vi "current monitor.vi"() -> ()   [LabVIEW 2010]
uses:
  <vilib>/Utility/file.llb/Write To Spreadsheet File (DBL).vi
  <userlib>/Nanonis Prog Interface V5/Nanonis Prog Interface.lvlib
panel:
  in  "Convert to nm/s?":bool caption="Spectrum Analyzer 2"
  out "Spectrum Analyzer 2":cluster{"f0":dbl, "df":dbl, "values":dbl[]}(graph)
  in  "Spectrum Analyzer2":bool caption="Spectrum Analyzer 2"
  out "error out":errorcluster
  in  "Path":path
  out "Spectrum Analyzer":cluster{"f0":dbl, "df":dbl, "values":dbl[]}(graph)
  out "Current (A)":sgl format="%#_6p"
  out "Current":cluster{"Current (A)":dbl, dbl}[](graph)
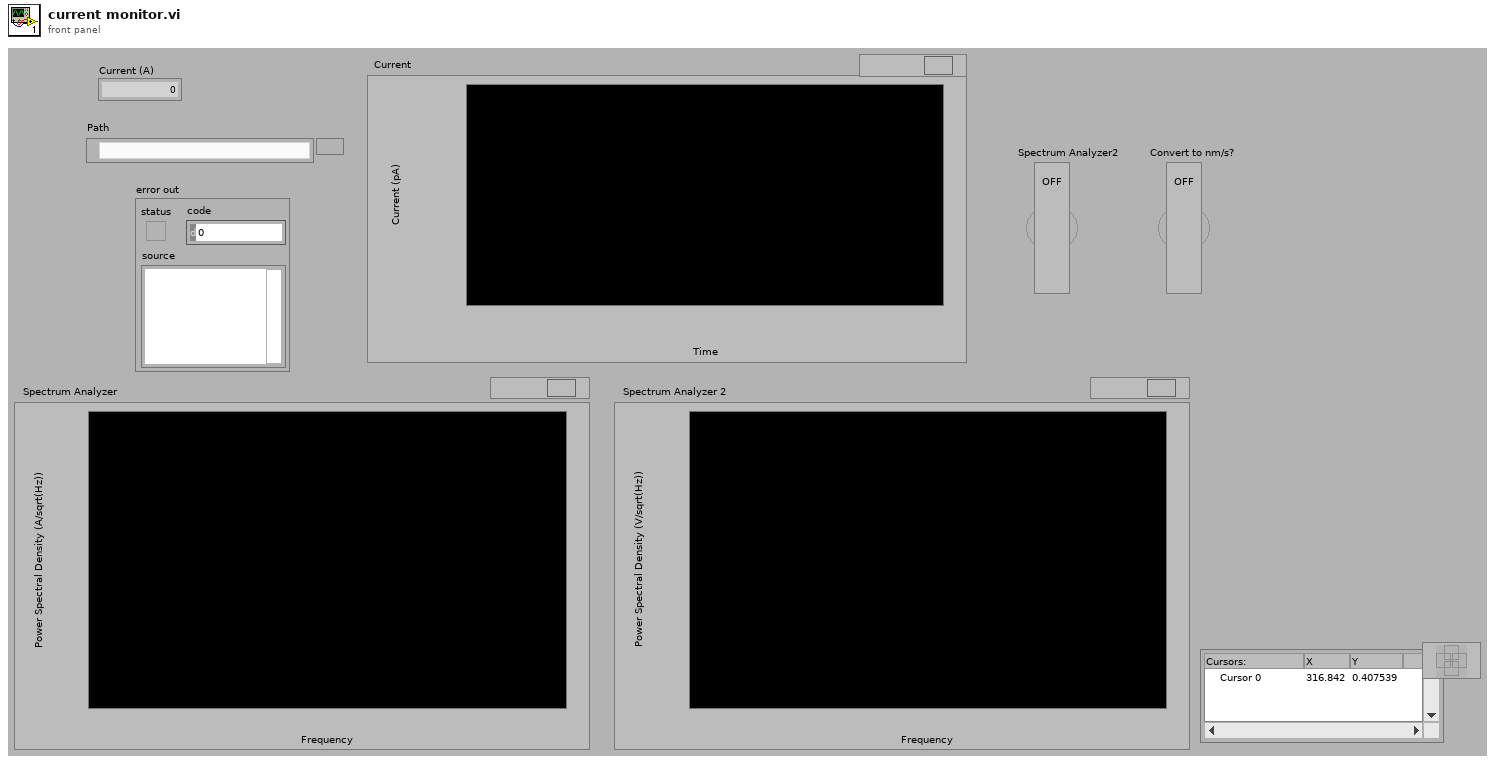
[diagram p1: front panel]
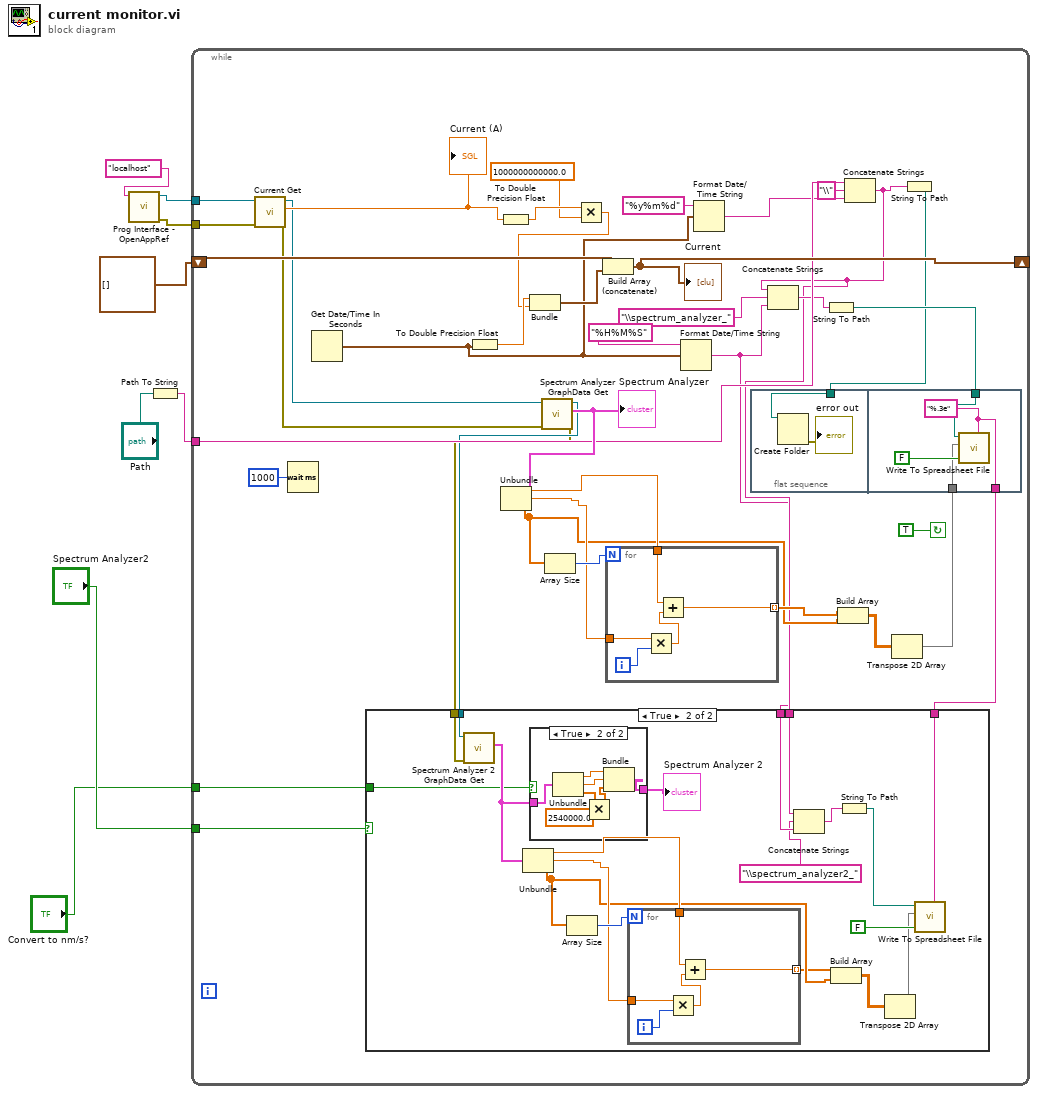
[diagram p0: block diagram]
diagram:
  n1 = call <userlib>:"Prog Interface - OpenAppRef.vi"("Machine name (local machine IP)"="localhost" ("machine name (localhost)")) -> ("Error out"=w7:errorcluster, "Application reference"=w8:refnum<vi>)  [unwired: 5 in]
  n2 = Path To String(path="Path") -> (string=w3:string)
  n3 = while {
    tunnel: w8 -> [w46]
    tunnel: w7 -> [w45]
    shift-right: [w42] -> _
    shift-left: cluster{dbl, dbl}[] [] -> [w43]
    tunnel: w3 -> [w28]
    tunnel: "Spectrum Analyzer2" -> [w13]
    tunnel: "Convert to nm/s?" -> [w9]
    stop <- TRUE continue-if-true
    n4 = call <userlib>:"Current Get.vi"("Error in (no error)"=w45, "Application ref in"=w46) -> ("Error out"=w35:errorcluster, "Current (A)"=w40:sgl, "Application ref out"=w36:refnum<vi>)  [unwired: 5 in]
    "Current (A)" <- w40
    n5 = Wait (ms)(milliseconds to wait=u32 1000) -> ()  [unwired: 1 out]
    n6 = Get Date/Time In Seconds() -> (seconds since 1Jan1904=w29:timestamp)
    n7 = To Double Precision Float(number=w29) -> (double precision float=w41:dbl)
    n8 = To Double Precision Float(number=w40) -> (double precision float=w39:dbl)
    n9 = call <userlib>:"Spectrum Analyzer GraphData Get.vi"("Error in (no error)"=w35, "Application ref in"=w36) -> ("Error out"=w14:errorcluster, "FFT data"=w33:cluster{"f0":dbl, "df":dbl, "values":dbl[]}, "Application ref out"=w15:refnum<vi>)  [unwired: 7 in]
    "Spectrum Analyzer" <- w33
    n10 = Unbundle(w33) -> ("f0"=w21:dbl, "df"=w20:dbl, "values"=w18:dbl[])
    n11 = Array Size(array=w18) -> (size(s)=w22:i32)
    n12 = Multiply(x=w39, y=1000000000000.0) -> (x*y=w38:dbl)
    n13 = Bundle(w41, w38) -> (w44:cluster{dbl, dbl})  [unwired: 1 in]
    n14 = Build Array (concatenate)(w43, w44) -> (w42:cluster{dbl, dbl}[])
    "Current" <- w42
    n15 = for {
      N: w22 -> [_]
      tunnel: w21 -> [w84]
      tunnel: w20 -> [w81]
      tunnel: [w80] -> w19 mode=indexing
      i -> [w82]
      n16 = Multiply(x=w81, y=w82) -> (x*y=w83:dbl)
      n17 = Add(x=w84, y=w83) -> (x+y=w80:dbl)
    }
    n18 = Format Date/Time String(time format string (%c)="%H%M%S", seconds (now)=w29) -> (date/time string=w11:string)  [unwired: 1 in]
    n19 = Format Date/Time String(time format string (%c)="%y%m%d", seconds (now)=w29) -> (date/time string=w26:string)  [unwired: 1 in]
    n20 = flat-sequence {
      tunnel: w27 -> [w86]
      tunnel: w31 -> [w88]
      tunnel: w16 -> [w89]
      tunnel: [w87] -> w10
      frame #0 {
        n21 = Create Folder(path (use dialog)=w86) -> (error out=→"error out":errorcluster)  [unwired: 2 in, 2 out]
      }
      frame #1 {
        w87 = "%.3e" ("format (%.3f)")
        n22 = call-poly <vilib>:"Write To Spreadsheet File.vi"("format (%.3f)"=w87, "append to file? (new file:F)"=FALSE, "2D data"=w89, "file path (dialog if empty)"=w88) -> ()  [unwired: 4 in, 1 out]
      }
    }
    n23 = Build Array(w19, w18) -> (w17:dbl[][])
    n24 = Concatenate Strings(w28, "\\" ("string"), w26) -> (w12:string)
    n25 = case shown="True" w13 {
      tunnel: w15 -> [_ w66]
      tunnel: w14 -> [_ w65]
      tunnel: w12 -> [_ w56]
      tunnel: w11 -> [_ w55]
      tunnel: w10 -> [_ w51]
      tunnel: w9 -> [_ w48]
      frame False {
      }
      frame True {
        n26 = call <userlib>:"Spectrum Analyzer 2 GraphData Get.vi"("Error in (no error)"=w65, "Application ref in"=w66) -> ("FFT data"=w50:cluster{"f0":dbl, "df":dbl, "values":dbl[]})  [unwired: 7 in, 2 out]
        n27 = Unbundle(w50) -> ("f0"=w63:dbl, "df"=w62:dbl, "values"=w60:dbl[])
        n28 = case shown="True" w48 {
          tunnel: w50 -> [w67 w74]
          tunnel: [w67 w73] -> w49
          frame False {
          }
          frame True {
            n29 = Unbundle(w74) -> ("f0"=w72:dbl, "df"=w71:dbl, "values"=w70:dbl[])
            n30 = Multiply(x=w70, y=2540000.0) -> (x*y=w69:dbl[])
            n31 = Bundle("f0"=w72, "df"=w71, w69) -> (w73:cluster{"f0":dbl, "df":dbl, dbl[]})  [unwired: 1 in]
          }
        }
        "Spectrum Analyzer 2" <- w49
        n32 = Array Size(array=w60) -> (size(s)=w64:i32)
        n33 = for {
          N: w64 -> [_]
          tunnel: w63 -> [w79]
          tunnel: w62 -> [w76]
          tunnel: [w75] -> w59 mode=indexing
          i -> [w77]
          n34 = Multiply(x=w76, y=w77) -> (x*y=w78:dbl)
          n35 = Add(x=w79, y=w78) -> (x+y=w75:dbl)
        }
        n36 = Concatenate Strings(w56, "\\spectrum_analyzer2_" ("string"), w55) -> (w52:string)
        n37 = Build Array(w59, w60) -> (w61:dbl[][])
        n38 = String To Path(string=w52) -> (path=w53:path)
        n39 = Transpose 2D Array(2D array=w61) -> (transposed array=w57:dbl[][])
        n40 = call-poly <vilib>:"Write To Spreadsheet File.vi"("format (%.3f)"=w51, "append to file? (new file:F)"=FALSE, "2D data"=w57, "file path (dialog if empty)"=w53) -> ()  [unwired: 4 in, 1 out]
      }
    }
    n41 = Concatenate Strings(w12, "\\spectrum_analyzer_" ("string"), w11) -> (w23:string)
    n42 = String To Path(string=w23) -> (path=w31:path)
    n43 = Transpose 2D Array(2D array=w17) -> (transposed array=w16:dbl[][])
    n44 = String To Path(string=w12) -> (path=w27:path)
  }
